vi "Scan.vi"(8 "error in":errorcluster, 11 "Local Data":T2) -> (0 "error out":errorcluster, 3 "Acquisition Scan":T1 {"Time Stamp" format="%<%x %.3X>T"})   [LabVIEW 2025, in "Instrument A.lvlib"]
uses:
  Controls/Local Data_Acquisition.ctl
  Instrument A.lvlib
  Controls/Acquisition Packet.ctl
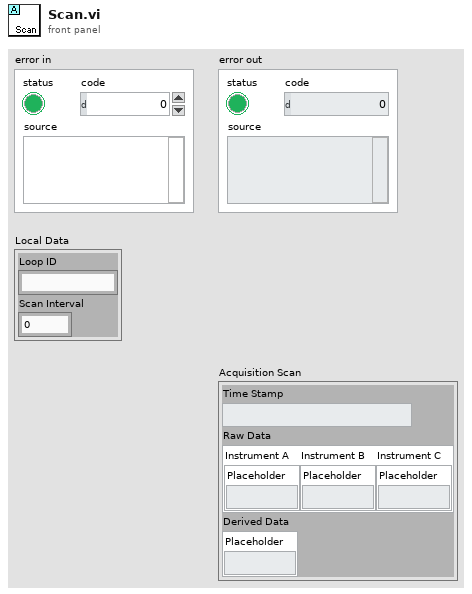
[diagram p1: front panel]
types:
  T1 = typedef "Acquisition Packet.ctl" = cluster{"Time Stamp":timestamp, "Raw Data":cluster{"Instrument A":cluster{"Placeholder":string}, "Instrument B":cluster{"Placeholder":string}, "Instrument C":cluster{"Placeholder":string}}, "Derived Data":cluster{"Placeholder":string}}
  T2 = typedef "Local Data_Acquisition.ctl" = cluster{"Loop ID":string, "Scan Interval":u32}
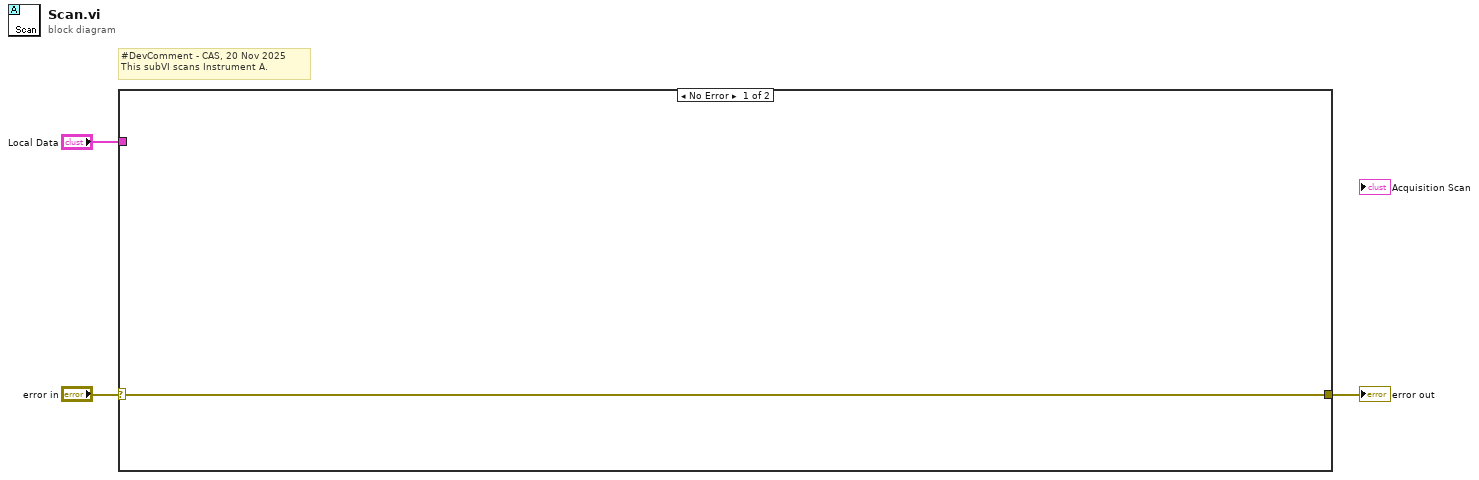
[diagram p0: block diagram]
diagram:
  # "#DevComment - CAS, 20 Nov 2025\nThis subVI scans Instrument A."
  n1 = case shown="No Error" "error in" {
    selector: "error in" -> [w4 w5]
    tunnel: [w4 w5] -> w2
    tunnel: "Local Data" -> [_ _]
    frame No Error {
    }
    frame Error {
    }
  }
  "error out" <- w2
